vi "Simple Read  Lock-in DAQ.vi"(7 "Initialize?":bool, 8 "error in (no error)":errorcluster, 9 "DAQ timeout, s":dbl=10.0 format="%0.2f", 10 "DAQ Task Array":refnum<k21>[](array[refnum]), 11 "Lock-in settings":T1={"Sine Frequency, Hz"=0.0, "Time constant, s"=0.12500000000000006, "Low-pass filter"=enum."No filtering", "Output representation"=enum."Real/Imaginary", "Phases, deg"=[], "Low-pass filter Order"=1, "Decimating factor"=1, "Samples to Read"=10000, "Post-filter decimation"=1, "Blocks to average"=1, "Trig delay, points"=0, "Harmonics per channel"=[], "Amplitude scale"=enum."RMS"} {"Time constant, s" format="%.1e"}) -> (0 "error out":errorcluster, 1 "Avg. signal(s)":dbl[](array[numeric]) format="%#_8e", 2 "DAQ Task Array Out":refnum<k21>[](array[refnum]), 3 "Lock-in settings out":T1={"Sine Frequency, Hz"=0.0, "Time constant, s"=0.12500000000000006, "Low-pass filter"=enum."No filtering", "Output representation"=enum."Real/Imaginary", "Phases, deg"=[], "Low-pass filter Order"=1, "Decimating factor"=1, "Samples to Read"=10000, "Post-filter decimation"=1, "Blocks to average"=1, "Trig delay, points"=0, "Harmonics per channel"=[], "Amplitude scale"=enum."RMS"} {"Time constant, s" format="%.1e"}, 4 "signal(s) out":dbl[][](array[numeric]), 5 "AvailSampPerChan":u32, 6 "Raw data":waveform(dbl)[](array[waveform]))   [LabVIEW 2020]
uses:
  Lockin Settings.ctl
  Harmonics per channel.ctl
  <vilib>/Waveform/WDTOps.llb/WDT Append Waveforms DBL.vi
  <vilib>/Waveform/WDTOps.llb/WDT Number of Waveform Samples DBL.vi
panel:
  out "number of samples":i32
  out "Waveform Graph":waveform(dbl)[](graph)
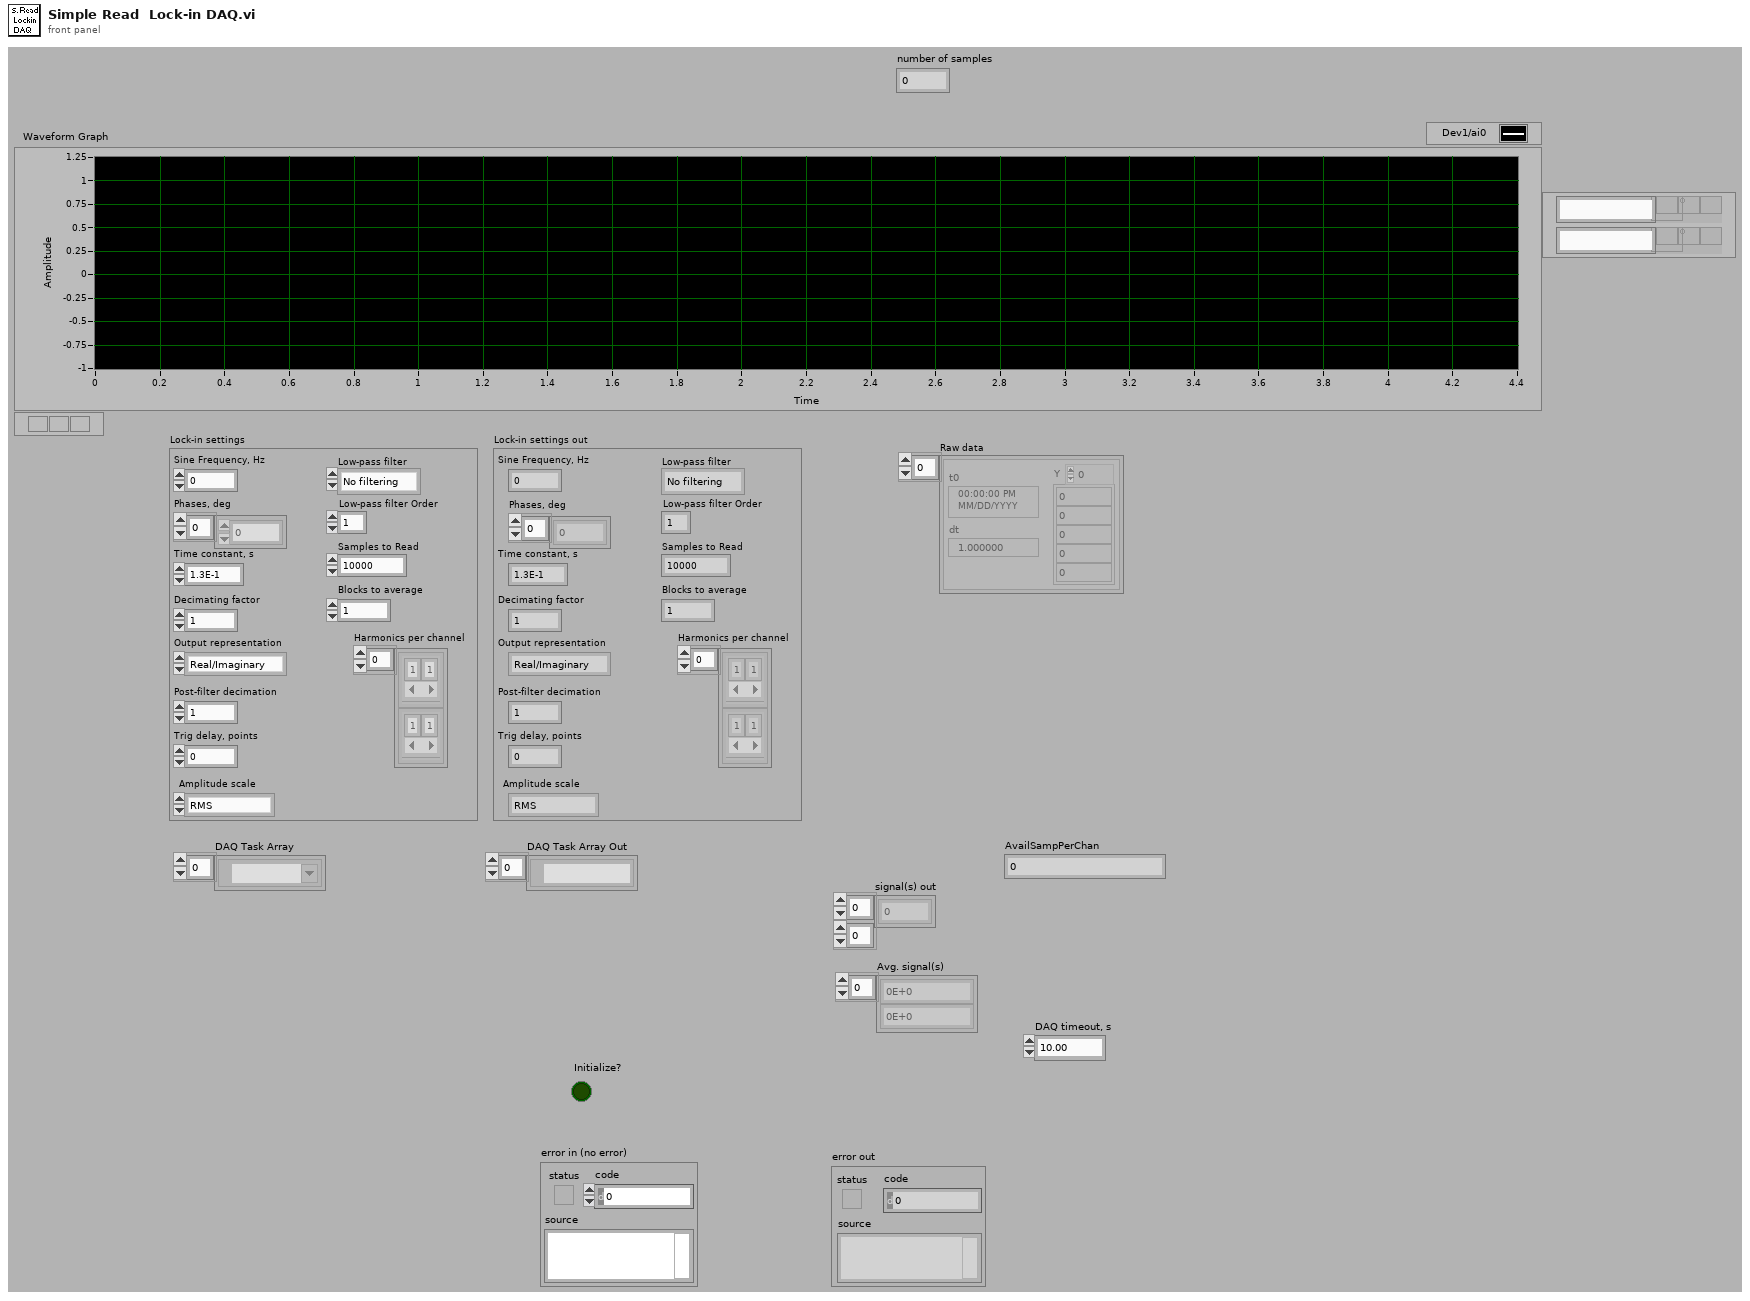
[diagram p1: front panel]
types:
  T1 = typedef "Lockin Settings.ctl" = cluster{"Sine Frequency, Hz":dbl, "Time constant, s":dbl, "Low-pass filter":enum16{"No filtering", "Butterworth", "Bessel"}, "Output representation":enum16{"Real/Imaginary", "Polar"}, "Phases, deg":dbl[], "Low-pass filter Order":i32, "Decimating factor":i32, "Samples to Read":i32, "Post-filter decimation":i32, "Blocks to average":i32, "Trig delay, points":i32, "Harmonics per channel":T2, "Amplitude scale":enum16{"Amplitude", "RMS", "Peak-to-Peak"}}
  T2 = typedef "Harmonics per channel.ctl" = cluster{"Harmonics":i32[]}[]
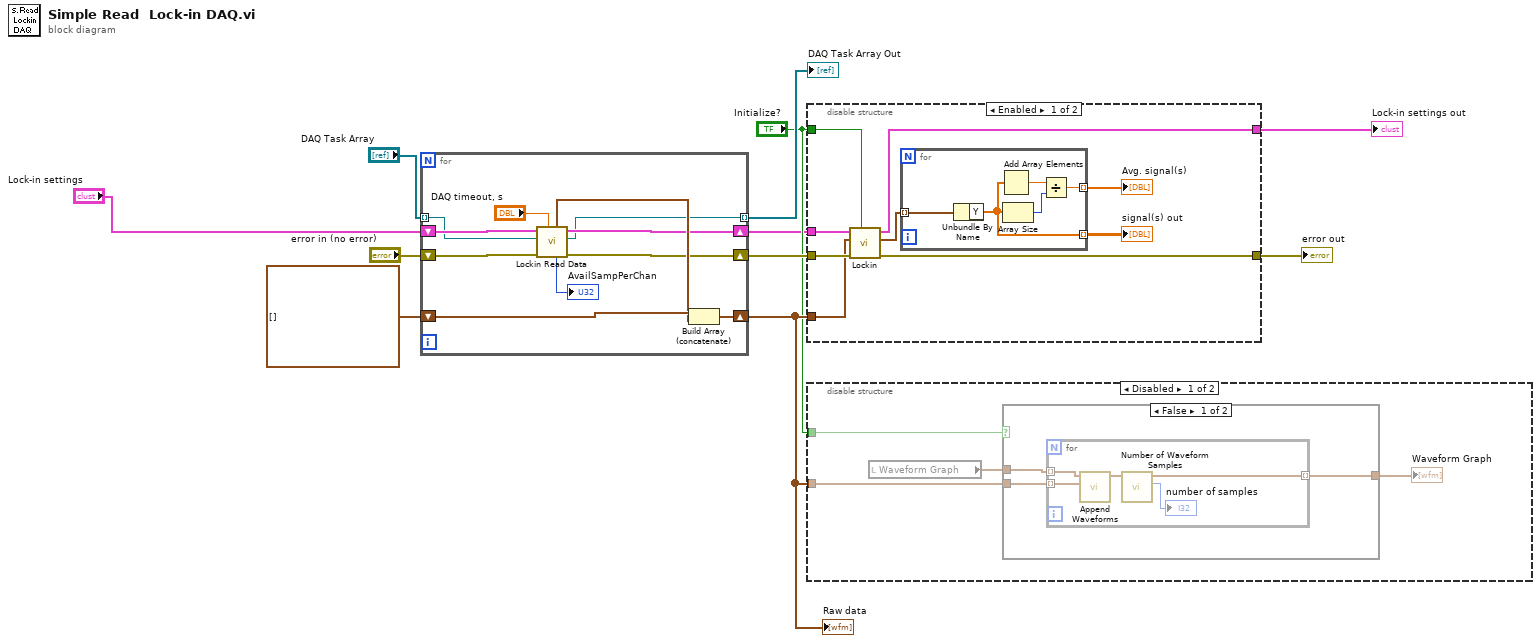
[diagram p0: block diagram]
diagram:
  n1 = for {
    tunnel: "DAQ Task Array" -> [w12] mode=indexing
    shift-right: [w22] -> w5
    shift-left: waveform(dbl)[] [] -> [w21]
    shift-right: [w16] -> w6
    shift-left: "error in (no error)" -> [w20]
    tunnel: [w13] -> w8 mode=indexing
    shift-right: [w14] -> w2
    shift-left: "Lock-in settings" -> [w15]
    n2 = call "Lockin Read Data.vi"("DAQ timeout, s"="DAQ timeout, s", "error in (no error)"=w20, "DAQ task"=w12, "Lock-in settings"=w15) -> ("error out"=w16:errorcluster, "task out"=w13:refnum<k21>, "Lock-in settings out"=w14:T1, "AvailSampPerChan"=→"AvailSampPerChan":u32, "data"=w18:waveform(dbl)[])  [unwired: 3 in]
    n3 = Build Array (concatenate)(w21, w18) -> (w22:waveform(dbl)[])
  }
  "DAQ Task Array Out" <- w8
  "Raw data" <- w5
  n4 = disable-structure shown="Enabled" {
    disable-tunnel: w2 -> [w25 _]
    disable-tunnel: [w30 w37] -> w10
    disable-tunnel: "Initialize?" -> [w24 _]
    disable-tunnel: w6 -> [w28 w37]
    disable-tunnel: w5 -> [w26 _]
    disable-tunnel: [w23 _] -> w1
    frame Enabled {
      n5 = call "Lockin.vi"("Initialize?"=w24, "error in (no error)"=w28, "data"=w26, "Lock-in settings"=w25) -> ("error out"=w30:errorcluster, "signal(s) out"=w27:waveform(dbl)[], "Lock-in settings out"=w23:T1)  [unwired: 5 in]
      n6 = for {
        tunnel: w27 -> [w36] mode=indexing
        tunnel: [w33] -> w31 mode=indexing
        tunnel: [w32] -> w29 mode=indexing
        n7 = Unbundle By Name(w36) -> ("Y"=w33:dbl[])
        n8 = Add Array Elements(numeric array=w33) -> (sum=w35:dbl)
        n9 = Array Size(array=w33) -> (size(s)=w34:i32)
        n10 = Divide(x=w35, y=w34) -> (x/y=w32:dbl)
      }
      "signal(s) out" <- w31
      "Avg. signal(s)" <- w29
    }
    frame Disabled {
    }
  }
  "error out" <- w10
  "Lock-in settings out" <- w1
  n11 = disable-structure shown="Disabled" {
    disable-tunnel: w5 -> [w40 _]
    disable-tunnel: "Initialize?" -> [w38 _]
    frame Disabled {
      n12 = local read "Waveform Graph"() -> (w41:waveform(dbl)[])
      n13 = case shown="False" w38 {
        tunnel: w41 -> [w44 _]
        tunnel: w40 -> [w43 w50]
        tunnel: [w42 w50] -> w39
        frame False {
          n14 = for {
            tunnel: w44 -> [w49] mode=indexing
            tunnel: w43 -> [w48] mode=indexing
            tunnel: [w46] -> w42 mode=indexing
            n15 = call-poly <vilib>:"Append Waveforms.vi"("waveform B"=w48, "waveform A"=w49) -> ("waveform out"=w47:waveform(dbl))  [unwired: 8 in, 1 out]
            n16 = call-poly <vilib>:"Number of Waveform Samples.vi"("waveform in"=w47) -> ("number of samples"=→"number of samples":i32, "waveform out"=w46:waveform(dbl))  [unwired: 8 in, 1 out]
          }
        }
        frame True {
        }
      }
      "Waveform Graph" <- w39
    }
    frame Enabled {
    }
  }
